vi "Generate BitfilePath.vi"() -> (0 "Bitfile path":path)   [LabVIEW 2019, in "FPGA Addon Adding a Channel Item.lvclass"]
uses:
  FPGA Addon Adding a Channel Item.lvclass
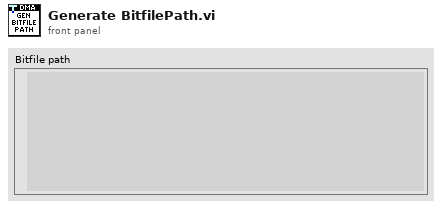
[diagram p1: front panel]
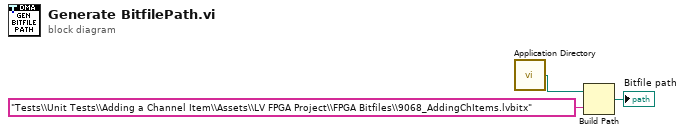
[diagram p0: block diagram]
diagram:
  n1 = call <vilib>:"Application Directory.vi"() -> ("Application Directory"=w3:path)
  n2 = Build Path(base path=w3, name or relative path="Tests\\Unit Tests\\Adding a Channel Item\\Assets\\LV FPGA Project\\FPGA Bitfiles\\9068_AddingChItems.lvbitx") -> (appended path=→"Bitfile path":path)
